vi "Create.vi"(8 "error in (no error)":errorcluster) -> (0 "error out":errorcluster, 3 "Event Registration Refnum":refnum<event-registration>)   [LabVIEW 2017, in "WebServiceImporter.lvlib" / "Main Panel.lvlib" / "Progress.lvlib" / "Events.lvlib"]
uses:
  <vilib>/Platform/WebService/Main Panel/Pages/Progress/Events/Events.lvlib
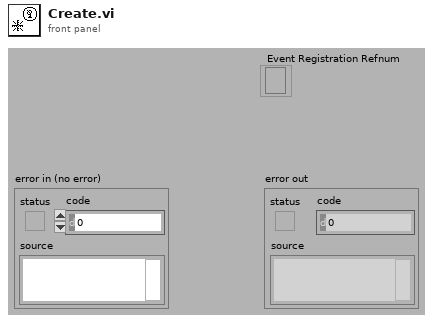
[diagram p1: front panel]
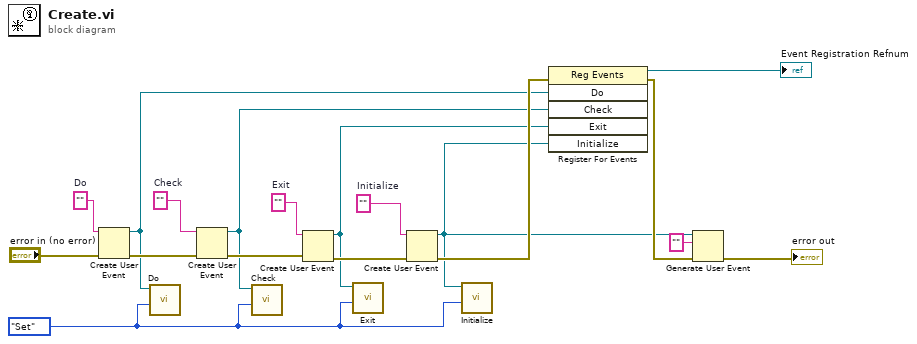
[diagram p0: block diagram]
diagram:
  w9 = ""  # Do
  w15 = ""  # Initialize
  w17 = ""  # Exit
  w1 = enum16{"Get", "Set"}."Set" ("Operation")
  w18 = ""  # Check
  n1 = Create User Event(user event datatype=w9, error in="error in (no error)") -> (user event=w2:refnum<user-event>, error out=w8:errorcluster)
  n2 = call <vilib>:"Do.vi"("Operation"=w1, "user event"=w2) -> ()  [unwired: 8 in, 2 out]
  n3 = Create User Event(user event datatype=w18, error in=w8) -> (user event=w5:refnum<user-event>, error out=w16:errorcluster)
  n4 = call <vilib>:"Check.vi"("Operation"=w1, "user event"=w5) -> ()  [unwired: 9 in, 1 out]
  n5 = Create User Event(user event datatype=w17, error in=w16) -> (user event=w6:refnum<user-event>, error out=w14:errorcluster)
  n6 = call <vilib>:"Exit.vi"("Operation"=w1, "user event"=w6) -> ()  [unwired: 8 in, 2 out]
  n7 = Create User Event(user event datatype=w15, error in=w14) -> (user event=w7:refnum<user-event>, error out=w13:errorcluster)
  n8 = call <vilib>:"Initialize.vi"("Operation"=w1, "user event"=w7) -> ()  [unwired: 9 in, 1 out]
  n9 = register-events(error in=w13, w2, w5, w6, w7) -> (reference out=→"Event Registration Refnum":refnum<event-registration>, error out=w11:errorcluster)  [unwired: 1 in]
  n10 = Generate User Event(user event=w7, event data cluster="" ("event data"), error in=w11) -> (error out=→"error out":errorcluster)  [unwired: 1 in, 1 out]
